vi "Day 4.vi"() -> ()   [LabVIEW 2018]
panel:
  out "Thermometer":dbl(slide) scale=0.0..100.0
  out "Warnings":string
  out "Very High":bool
  in  "Slide":dbl(slide) scale=0.0..100.0
  out "?":bool
  out "?":bool
  out "?":bool
  in  "Boolean":bool
  out "Boolean 2":bool
  out "String":string
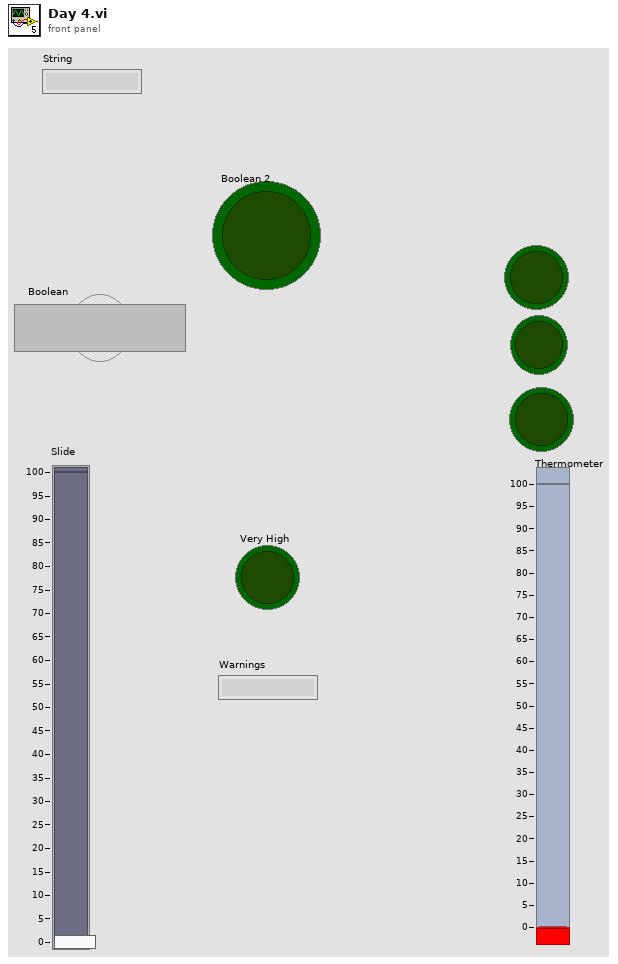
[diagram p1: front panel]
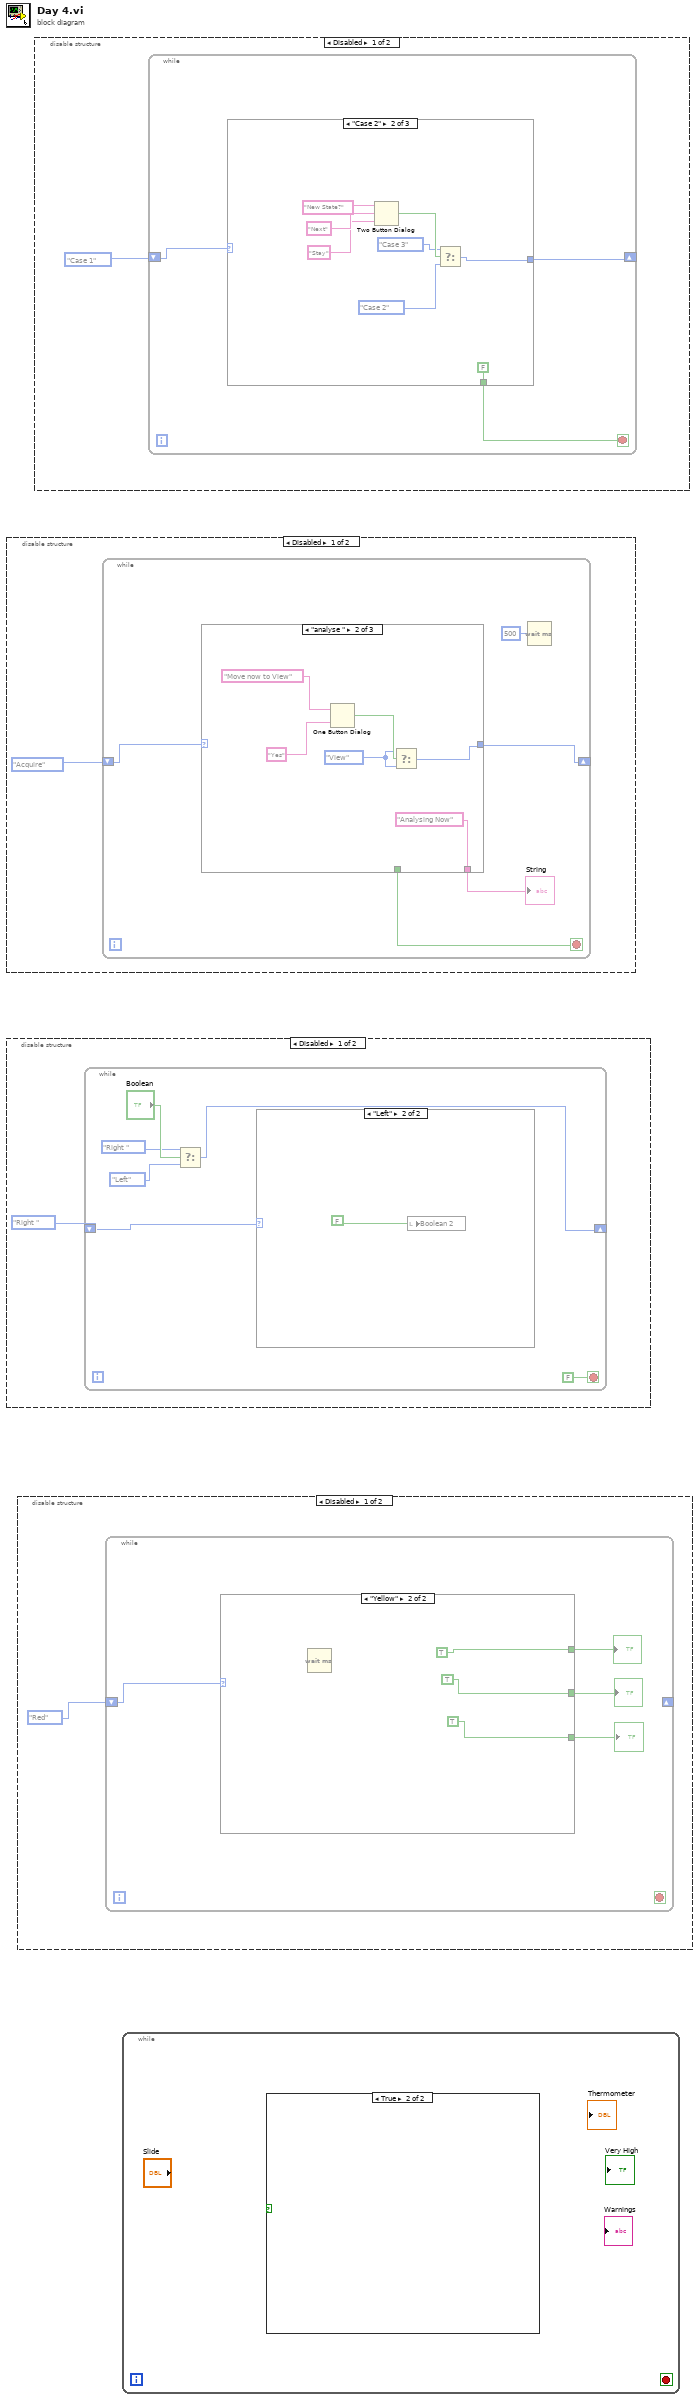
[diagram p0: block diagram]
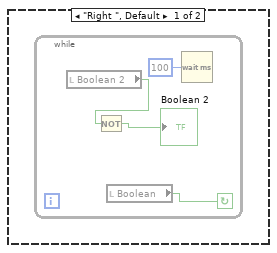
[diagram p5: hidden frame]
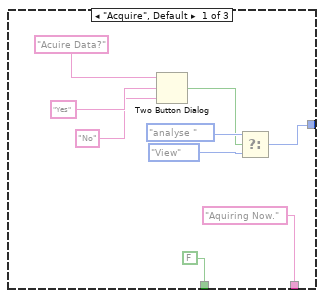
[diagram p7: hidden frame]
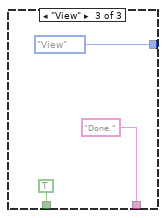
[diagram p8: hidden frame]
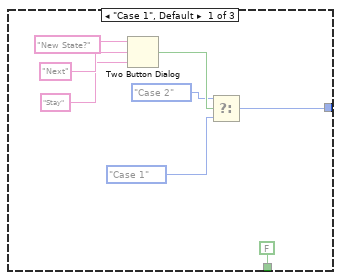
[diagram p10: hidden frame]
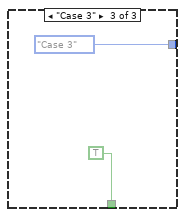
[diagram p11: hidden frame]
diagram:
  n1 = disable-structure shown="Disabled" {
    frame Disabled {
      n2 = while {
        shift-right: [w3] -> _
        shift-left: enum16{"Right ", "Left"}."Right " -> [w7]
        stop <- FALSE stop-if-true
        n3 = Select(t=enum16{"Right ", "Left"}."Right ", s="Boolean", f=enum16{"Right ", "Left"}."Left") -> (s? t:f=w3:enum16{"Right ", "Left"})
        n4 = case shown="\"Left\"" w7 {
          frame "Right ", Default {
            n5 = while {
              stop <- w11 continue-if-true
              n6 = local read "Boolean 2"() -> (w9:bool)
              n7 = Not(x=w9) -> (.not. x?=→"Boolean 2":bool)
              n8 = local read "Boolean"() -> (w11:bool)
              n9 = Wait (ms)(milliseconds to wait=u32 100) -> ()  [unwired: 1 out]
            }
          }
          frame "Left" {
            n10 = local write "Boolean 2"(FALSE) -> ()
          }
        }
      }
    }
    frame Enabled {
    }
  }
  n11 = disable-structure shown="Disabled" {
    frame Disabled {
      n12 = while {
        shift-right: [w18] -> _
        shift-left: enum16{"Acquire", "analyse ", "View", ""}."Acquire" -> [w17]
        stop <- w16 stop-if-true
        n13 = case shown="\"analyse \"" w17 {
          tunnel: [w24 w31 enum16{"Acquire", "analyse ", "View", ""}."View"] -> w18
          tunnel: [FALSE _ TRUE] -> w16
          tunnel: ["Aquiring Now." "Analysing Now" "Done."] -> w15
          frame "Acquire", Default {
            n14 = Two Button Dialog(message="Acuire Data?", 1:"No" ("F button name (\"Cancel\")"), 2:"Yes" ("T button name (\"OK\")")) -> (T button?=w20:bool)
            n15 = Select(t=enum16{"Acquire", "analyse ", "View", ""}."analyse ", s=w20, f=enum16{"Acquire", "analyse ", "View", ""}."View") -> (s? t:f=w24:enum16{"Acquire", "analyse ", "View", ""})
          }
          frame "analyse " {
            w29 = enum16{"Acquire", "analyse ", "View", ""}."View"
            n16 = One Button Dialog(message="Move now to View", button name ("OK")="Yes" ("F button name (\"Cancel\")")) -> (true=w30:bool)
            n17 = Select(t=w29, s=w30, f=w29) -> (s? t:f=w31:enum16{"Acquire", "analyse ", "View", ""})
          }
          frame "View" {
          }
        }
        "String" <- w15
        n18 = Wait (ms)(milliseconds to wait=u32 500) -> ()  [unwired: 1 out]
      }
    }
    frame Enabled {
    }
  }
  n19 = disable-structure shown="Disabled" {
    frame Disabled {
      n20 = while {
        shift-right: _ -> [_]
        shift-left: enum16{"Red", "Yellow", "Green"}."Red" -> [w41]
        stop <- _ stop-if-true
        n21 = case shown="\"Yellow\"" w41 {
          tunnel: [_ TRUE] -> w40
          tunnel: [_ TRUE] -> w39
          tunnel: [_ TRUE] -> w38
          frame "Red", Default {
          }
          frame "Yellow" {
            n22 = Wait (ms)() -> ()  [unwired: 1 in, 1 out]
          }
        }
        "?" <- w40
        "?" <- w39
        "?" <- w38
      }
    }
    frame Enabled {
    }
  }
  n23 = disable-structure shown="Disabled" {
    frame Disabled {
      n24 = while {
        shift-right: [w47] -> _
        shift-left: enum16{"Case 1", "Case 2", "Case 3"}."Case 1" -> [w48]
        stop <- w46 stop-if-true
        n25 = case shown="\"Case 2\"" w48 {
          tunnel: [w50 w58 enum16{"Case 1", "Case 2", "Case 3"}."Case 3"] -> w47
          tunnel: [FALSE FALSE TRUE] -> w46
          frame "Case 1", Default {
            n26 = Two Button Dialog(message="New State?", 1:"Stay" ("F button name (\"Cancel\")"), 2:"Next" ("T button name (\"OK\")")) -> (T button?=w53:bool)
            n27 = Select(t=enum16{"Case 1", "Case 2", "Case 3"}."Case 2", s=w53, f=enum16{"Case 1", "Case 2", "Case 3"}."Case 1") -> (s? t:f=w50:enum16{"Case 1", "Case 2", "Case 3"})
          }
          frame "Case 2" {
            n28 = Two Button Dialog(message="New State?", 1:"Stay" ("F button name (\"Cancel\")"), 2:"Next" ("T button name (\"OK\")")) -> (T button?=w61:bool)
            n29 = Select(t=enum16{"Case 1", "Case 2", "Case 3"}."Case 3", s=w61, f=enum16{"Case 1", "Case 2", "Case 3"}."Case 2") -> (s? t:f=w58:enum16{"Case 1", "Case 2", "Case 3"})
          }
          frame "Case 3" {
          }
        }
      }
    }
    frame Enabled {
    }
  }
  n30 = while {
    stop <- _ stop-if-true
    n31 = case shown="True" {
      selector: _ -> [_ _]
      frame False {
      }
      frame True {
      }
    }
  }
